vi "test get from map as type.vi"() -> (1 "pass?":bool)   [LabVIEW 2019, in "ANODE Tests.lvlib"]
uses:
  my_type.ctl
  b7fdc737-810d-476c-803f-87d92304fadd.vi
  7fb67aad-f021-4248-8772-102f8fa4be12.vi
  03525885-fed1-44f0-abe8-b2b06852e5b1.vi
  eb1a332b-77f4-454b-9d65-ac763f45a6a6.vi
  6fdd71bf-bd25-4e1a-bc78-942183a96767.vi
  209f202e-6f5e-4ae7-91fa-58a3fdf974fc.vi
  15cceecd-e535-48b2-a859-5fa44f02509e.vi
  98d83769-089f-491f-aeb6-b46676a4fedc.vi
  7c66440c-c52d-4b3f-ad65-0164ab6378dc.vi
  b7fdc737-810d-476c-803f-87d92304fadd.vi/98980545-f0ee-459a-bc28-370193a87d2d.vi
  7fb67aad-f021-4248-8772-102f8fa4be12.vi/d86fdfde-6721-43bd-a64a-dcad4e61a4d7.vi
  7fb67aad-f021-4248-8772-102f8fa4be12.vi/4385d2f5-54b6-4bca-9c3c-d04521fe82b3.vi
  03525885-fed1-44f0-abe8-b2b06852e5b1.vi/956e9c22-915e-414c-90e9-684a0a93f871.vi
  03525885-fed1-44f0-abe8-b2b06852e5b1.vi/72ed93e5-0e6a-4db5-8097-6b846e804a79.vi
  eb1a332b-77f4-454b-9d65-ac763f45a6a6.vi/b38c5c1a-58e6-416f-8dc9-2feacd7a40b8.vi
  eb1a332b-77f4-454b-9d65-ac763f45a6a6.vi/5352505b-127c-4708-800e-524fa1aa54b4.vi
  6fdd71bf-bd25-4e1a-bc78-942183a96767.vi/20b4c8ce-dfee-49cf-8c79-668ff8617ffc.vi
  6fdd71bf-bd25-4e1a-bc78-942183a96767.vi/16ae8aaa-e8c1-422b-9e79-d2d0f5b536ca.vi
  209f202e-6f5e-4ae7-91fa-58a3fdf974fc.vi/891e1dc1-9a90-47c0-a89d-c43933cb2a71.vi
  15cceecd-e535-48b2-a859-5fa44f02509e.vi/6eda0150-bf65-4d6a-8b46-fcf438626008.vi
  15cceecd-e535-48b2-a859-5fa44f02509e.vi/08370c18-55ea-4a28-805c-5173874a83c8.vi
  98d83769-089f-491f-aeb6-b46676a4fedc.vi/7691b878-0380-49e2-81ad-35b576de774c.vi
  98d83769-089f-491f-aeb6-b46676a4fedc.vi/9f5bc0bd-beb2-4cc8-b30d-9bfdec5def76.vi
  <vilib>/Utility/error.llb/Clear Errors.vi
  7c66440c-c52d-4b3f-ad65-0164ab6378dc.vi/30bb4909-7cc7-4b2a-8850-3e982f0a11b8.vi
  ANODE Tests.lvlib
panel:
  out "my_type":bool
  out "int arry pass?":bool
  out "sgl arry pass?":bool
  out "path pass?":bool
  out "U64 pass?":bool
  out "I32 pass?":bool
  out "U32 pass?":bool
  out "double pass?":bool
  out "string pass?":bool
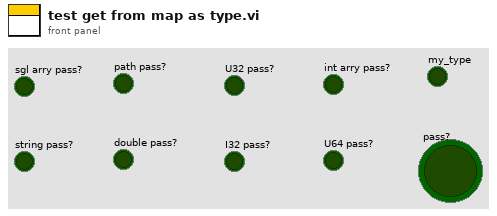
[diagram p1: front panel]
types:
  T1 = typedef "ANODE Tests.lvlib/my_type.ctl" = enum16{"test", "foo"}
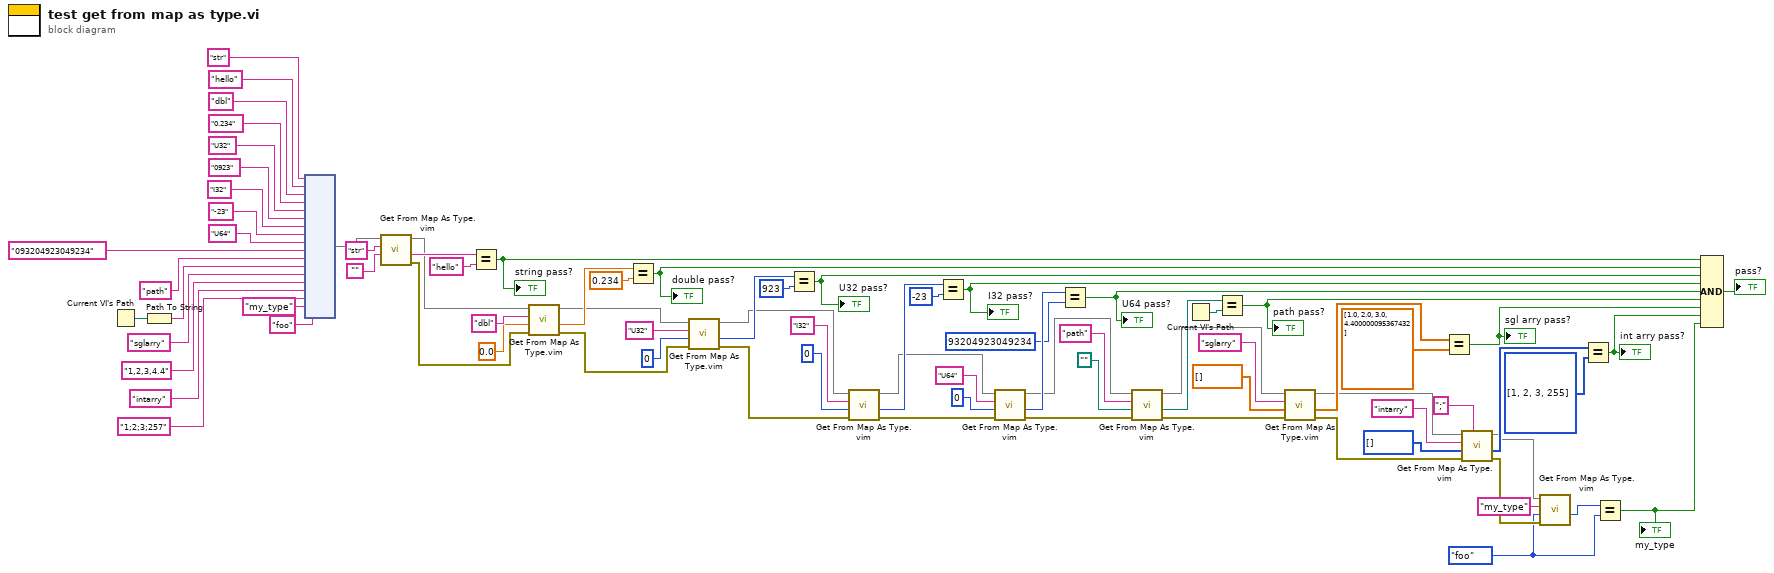
[diagram p0: block diagram]
diagram:
  w1 = my_type."foo" ("my_type")
  n1 = Current VI's Path() -> (path=w71:path)
  n2 = Path To String(path=w71) -> (string=w70:string)
  n3 = node("str", "hello", "dbl", "0.234", "U32", "0923", "I32", "-23", "U64", "093204923049234", "path", w70, "sglarry", "1,2,3,4.4", "intarry", "1;2;3;257", "my_type" ("key"), "foo" ("value")) -> (w65:map{string, string})
  n4 = call "Get From Map As Type.vim"("default"="", "key"="str", "map in"=w65) -> ("error out"=w30:errorcluster, "value"=w62:string, "map out (unchanged)"=w60:map{string, string})  [unwired: 5 in, 1 out]
  n5 = Equal?(x=w62, y="hello") -> (x = y?=w17:bool)
  "string pass?" <- w17
  n6 = call "Get From Map As Type.vim"("error in (no error)"=w30, "default"=0.0, "key"="dbl", "map in"=w60) -> ("error out"=w29:errorcluster, "value"=w57:dbl, "map out (unchanged)"=w52:map{string, string})  [unwired: 4 in, 1 out]
  n7 = Equal?(x=w57, y=0.234) -> (x = y?=w16:bool)
  "double pass?" <- w16
  n8 = call "Get From Map As Type.vim"("error in (no error)"=w29, "default"=u32 0 ("y"), "key"="U32", "map in"=w52) -> ("error out"=w28:errorcluster, "value"=w54:u32, "map out (unchanged)"=w46:map{string, string})  [unwired: 4 in, 1 out]
  n9 = Equal?(x=w54, y=u32 923) -> (x = y?=w15:bool)
  "U32 pass?" <- w15
  n10 = call "Get From Map As Type.vim"("error in (no error)"=w28, "default"=0 ("y"), "key"="I32", "map in"=w46) -> ("error out"=w27:errorcluster, "value"=w49:i32, "map out (unchanged)"=w41:map{string, string})  [unwired: 4 in, 1 out]
  n11 = Equal?(x=w49, y=-23) -> (x = y?=w14:bool)
  "I32 pass?" <- w14
  n12 = call "Get From Map As Type.vim"("error in (no error)"=w27, "default"=u64 0 ("y"), "key"="U64", "map in"=w41) -> ("error out"=w26:errorcluster, "value"=w43:u64, "map out (unchanged)"=w40:map{string, string})  [unwired: 4 in, 1 out]
  n13 = Equal?(x=w43, y=u64 93204923049234) -> (x = y?=w13:bool)
  "U64 pass?" <- w13
  n14 = call "Get From Map As Type.vim"("error in (no error)"=w26, "default"=path "", "key"="path", "map in"=w40) -> ("error out"=w25:errorcluster, "value"=w37:path, "map out (unchanged)"=w35:map{string, string})  [unwired: 4 in, 1 out]
  n15 = Current VI's Path() -> (path=w36:path)
  n16 = Equal?(x=w37, y=w36) -> (x = y?=w12:bool)
  "path pass?" <- w12
  n17 = call "Get From Map As Type.vim"("error in (no error)"=w25, "default"=sgl[] [], "key"="sglarry", "map in"=w35) -> ("error out"=w24:errorcluster, "value"=w32:sgl[], "map out (unchanged)"=w23:map{string, string})  [unwired: 4 in, 1 out]
  n18 = Equal?(x=w32, y=sgl[] [1.0, 2.0, 3.0, 4.4]) -> (x = y?=w11:bool)
  "sgl arry pass?" <- w11
  n19 = call "Get From Map As Type.vim"("array delimeter (,)"=";", "error in (no error)"=w24, "default"=u8[] [], "key"="intarry", "map in"=w23) -> ("error out"=w6:errorcluster, "value"=w19:u8[], "map out (unchanged)"=w5:map{string, string})  [unwired: 3 in, 1 out]
  n20 = call "Get From Map As Type.vim"("error in (no error)"=w6, "default"=w1, "key"="my_type", "map in"=w5) -> ("value"=w3:T1)  [unwired: 4 in, 3 out]
  n21 = Equal?(x=w19, y=u8[] [1, 2, 3, 255]) -> (x = y?=w10:bool)
  "int arry pass?" <- w10
  n22 = Equal?(x=w3, y=w1) -> (x = y?=w2:bool)
  "my_type" <- w2
  n23 = Compound Arithmetic op=AND(w17, w16, w15, w14, w13, w12, w11, w10, w2) -> (→"pass?":bool)
